vi "TrackCircle.vi"(3 "Debug":bool, 4 "Track":bool, 5 "Mono Image In 2":T3, 6 "Color Image In":T3) -> (0 "Curves":T1[](array[typedef]) {"Points"."Y" format="%.2f"; "Points"."X" format="%.2f"}, 1 "Circles":i32, 2 "ColorImage Out":T3)   [LabVIEW 2017]
uses:
  <vilib>/vision/Image Controls.llb/IMAQ Image.ctl
  <vilib>/vision/Shape Detection.llb/ShapeDetectionMatchOptions.ctl
  <vilib>/vision/Pattern Matching.llb/IMAQ Match Range Setting.ctl
  <vilib>/vision/Pattern Matching.llb/IMAQ Curve Parameters.ctl
  <vilib>/vision/Analysis.llb/IMAQ ExtractCurvesCurve.ctl
  <vilib>/vision/NI_Vision_Development_Module.lvlib
panel:
  out "Circles":T2(array[cluster]) {"Position"."Y" format="%.2f"; "Position"."X" format="%.2f"}
  in  "Minimum match score":dbl=600.0
  in  "Curve Parameters":T4={"Extraction Mode"=0, "Edge Threshold"=50, "Edge Filter Size"=1, "Min Length"=25, "Row Search Step Size"=15, "Col Search Step Size"=15, "Max Endpoint Gap"=10, "Closed"=FALSE, "Subpixel"=FALSE} {"Extraction Mode" items=["Normal", "Uniform Regions"]; "Edge Filter Size" items=["Fine", "Normal", "Contour Tracing"]; "Max Endpoint Gap" min=0; "Col Search Step Size" min=1 max=255 step=1; "Row Search Step Size" min=1 max=255 step=1; "Min Length" min=0; "Edge Threshold" min=1 max=350 step=1}
  in  "Match Options":T5={"Rotation"=FALSE, "Scale"=FALSE, "Occlusion"=TRUE, "Range Settings"=[{"Match Constraints"=2, "Min"=0.0, "Max"=40.0}]} {"Range Settings"."Max" format="%.2f"; "Range Settings"."Min" format="%.2f"; "Range Settings"."Match Constraints" items=["Rotation Angle (degrees)", "Scale Factor (%)", "Occlusion (%)"]}
  in  "Circle Descriptor":cluster{"Min Radius":dbl, "Max Radius":dbl}={"Min Radius"=25.0, "Max Radius"=100.0}
  # "Range"
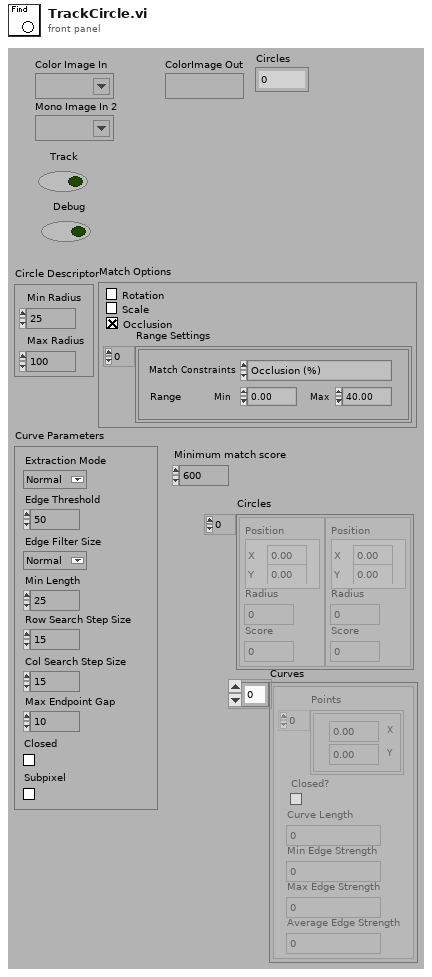
[diagram p1: front panel]
types:
  T1 = typedef "IMAQ ExtractCurvesCurve.ctl" = cluster{"Points":cluster{"X":dbl, "Y":dbl}[], "Closed?":bool, "Curve Length":dbl, "Min Edge Strength":dbl, "Max Edge Strength":dbl, "Average Edge Strength":dbl}
  T2 = cluster{"Position":cluster{"X":sgl, "Y":sgl}, "Radius":dbl, "Score":dbl}[]
  T3 = typedef "IMAQ Image.ctl" = refnum<image>
  T4 = typedef "IMAQ Curve Parameters.ctl" = cluster{"Extraction Mode":u32, "Edge Threshold":i32, "Edge Filter Size":u32, "Min Length":i32, "Row Search Step Size":i32, "Col Search Step Size":i32, "Max Endpoint Gap":i32, "Closed":bool, "Subpixel":bool}
  T5 = typedef "ShapeDetectionMatchOptions.ctl" = cluster{"Rotation":bool, "Scale":bool, "Occlusion":bool, "Range Settings":T6[]}
  T6 = typedef "IMAQ Match Range Setting.ctl" = cluster{"Match Constraints":u32, "Min":dbl, "Max":dbl}
  T7 = cluster{"Global Rectangle":i32[], "Contours":cluster{"ID":enum32{"External", "Internal"}, "Type":u32, "Coordinates":i32[]}[]}
  T8 = cluster{"Desired Font (Application)":enum16{"User-specified Font", "Application Font", "System Font", "Dialog Font"}, "[User-specified Font]":cluster{"Font Name":string, "Size":i16, "Strikeout?":bool, "Italic?":bool, "Underline?":bool, "Outline?":bool, "Shadow?":bool, "Bold?":bool, "Rotation Angle":dbl}, "Horizontal Alignment":i16, "Vertical Alignment":i16}
  T9 = typedef "IMAQ Rectangle" = cluster{"Left":i32, "Top":i32, "Right":i32, "Bottom":i32, "Rotation":dbl}
  T10 = typedef "ROI Descriptor" = cluster{"Global Rectangle":i32[], "Contours":cluster{"ID":enum32{"External", "Internal"}, "Type":u32, "Coordinates":i32[]}[]}
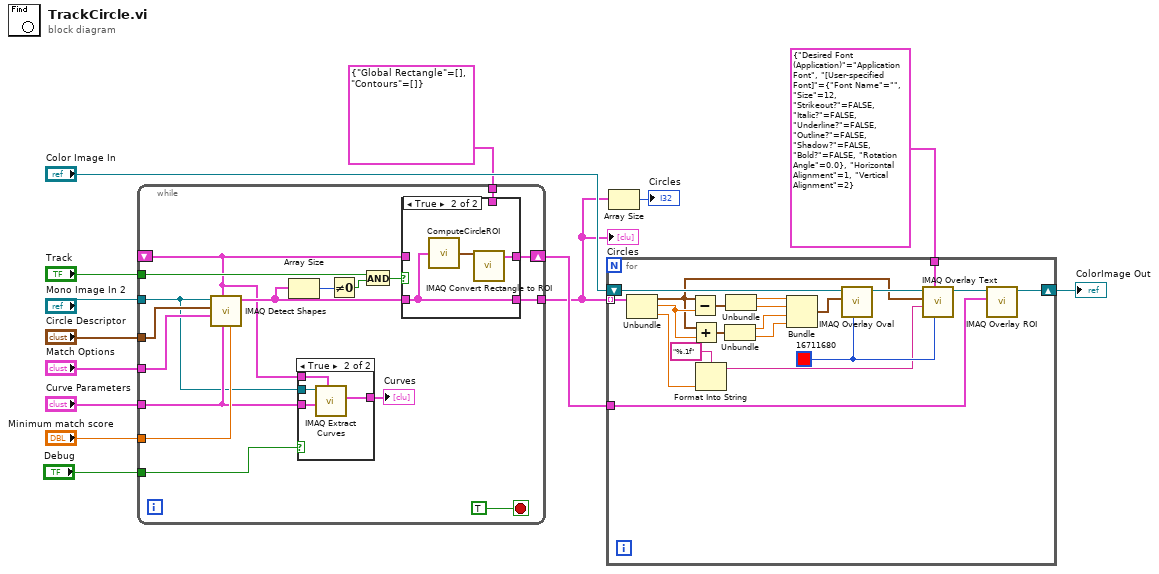
[diagram p0: block diagram]
diagram:
  n1 = while {
    tunnel: [w27] -> w3
    tunnel: "Circle Descriptor" -> [w31]
    tunnel: "Match Options" -> [w30]
    tunnel: "Curve Parameters" -> [w19]
    tunnel: "Minimum match score" -> [w29]
    tunnel: "Mono Image In 2" -> [w18]
    shift-right: [w26] -> w4
    shift-left: _ -> [w17]
    tunnel: "Track" -> [w28]
    tunnel: T7 {"Global Rectangle"=[], "Contours"=[]} ("ROI Descriptor") -> [w25]
    tunnel: "Debug" -> [w16]
    stop <- TRUE stop-if-true
    n2 = call-poly "IMAQ Detect Shapes"("Minimum match score"=w29, "Curve Parameters"=w19, "ROI Descriptor"=w17, "Match Options"=w30, "Circle Descriptor"=w31, "Image"=w18) -> ("Circles"=w22:T2)  [unwired: 3 in, 2 out]
    n3 = Array Size(array=w22) -> (size(s)=w21:i32)
    n4 = case shown="True" w16 {
      tunnel: w19 -> [_ w35]
      tunnel: w18 -> [_ w34]
      tunnel: w17 -> [_ w33]
      tunnel: [_ w32] -> w15
      frame False {
      }
      frame True {
        n5 = call "IMAQ Extract Curves"("ROI Descriptor"=w33, "Curve Parameters"=w35, "Image"=w34) -> ("Curves"=w32:T1[])  [unwired: 6 in, 2 out]
      }
    }
    "Curves" <- w15
    n6 = Not Equal To 0?(x=w21) -> (x != 0?=w20:bool)
    n7 = And(x=w28, y=w20) -> (x .and. y?=w23:bool)
    n8 = case shown="True" w23 {
      tunnel: w17 -> [_ _]
      tunnel: w22 -> [w37 w39]
      tunnel: [w37 w39] -> w27
      tunnel: [w36 w40] -> w26
      tunnel: w25 -> [w36 _]
      frame False {
      }
      frame True {
        n9 = call <vilib>:"ComputeCircleROI.vi"("Circles"=w39) -> ("Rectangle"=w38:T9)
        n10 = call "IMAQ Convert Rectangle to ROI"("Rectangle"=w38) -> ("ROI Descriptor"=w40:T10)  [unwired: 8 in, 1 out]
      }
    }
  }
  "Circles" <- w3
  n11 = for {
    shift-right: [w42] -> w14
    shift-left: "Color Image In" -> [w60]
    tunnel: w3 -> [w59] mode=indexing
    tunnel: T8 {"Desired Font (Application)"=enum."Application Font", "[User-specified Font]"={"Font Name"="", "Size"=12, "Strikeout?"=FALSE, "Italic?"=FALSE, "Underline?"=FALSE, "Outline?"=FALSE, "Shadow?"=FALSE, "Bold?"=FALSE, "Rotation Angle"=0.0}, "Horizontal Alignment"=1, "Vertical Alignment"=2} ("Font, Size & Style") -> [w49]
    tunnel: w4 -> [w41]
    w51 = u32 16711680 ("Color")
    n12 = Unbundle(w59) -> ("Position"=w46:cluster{"X":sgl, "Y":sgl}, "Radius"=w58:dbl, "Score"=w48:dbl)
    n13 = Subtract(x=w46, y=w58) -> (x-y=w57:cluster{"X":dbl, "Y":dbl})
    n14 = Add(x=w46, y=w58) -> (x+y=w56:cluster{"X":dbl, "Y":dbl})
    n15 = Format Into String(format string="%.1f", w48) -> (resulting string=w47:string)  [unwired: 2 in, 1 out]
    n16 = Unbundle(w56) -> ("X"=w53:dbl, "Y"=w52:dbl)
    n17 = Unbundle(w57) -> ("X"=w55:dbl, "Y"=w54:dbl)
    n18 = Bundle("X"=w55, "Y"=w54, "X"=w53, "Y"=w52) -> (w45:cluster{"X":dbl, "Y":dbl, "X":dbl, "Y":dbl})  [unwired: 1 in]
    n19 = call "IMAQ Overlay Oval"("Color"=w51, "Bounding Rectangle"=w45, "Image"=w60) -> ("Image Out"=w50:T3)  [unwired: 7 in, 1 out]
    n20 = call "IMAQ Overlay Text"("Text Color (black)"=w51, "Font, Size & Style"=w49, "String"=w47, "Origin"=w46, "Image"=w50) -> ("Image Out"=w43:T3)  [unwired: 5 in, 1 out]
    n21 = call "IMAQ Overlay ROI"("ROI Descriptor"=w41, "Image"=w43) -> ("Image Out"=w42:T3)  [unwired: 8 in, 1 out]
  }
  "ColorImage Out" <- w14
  n22 = Array Size(array=w3) -> (size(s)=→"Circles":i32)
